vi "OverlayFittedCircle.vi"(10 "Circle time series":dbl[][](array[numeric]), 11 "Image":T1) -> (3 "Image Out":T1)   [LabVIEW 2013]
uses:
  <vilib>/vision/Image Controls.llb/IMAQ Image.ctl
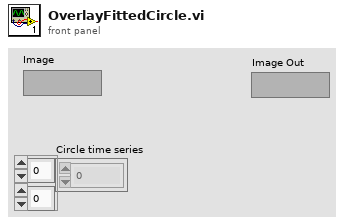
[diagram p1: front panel]
types:
  T1 = typedef "IMAQ Image.ctl" = refnum<image>
  T2 = cluster{"[0]":i32, "[1]":i32, "[2]":i32, "[3]":i32}
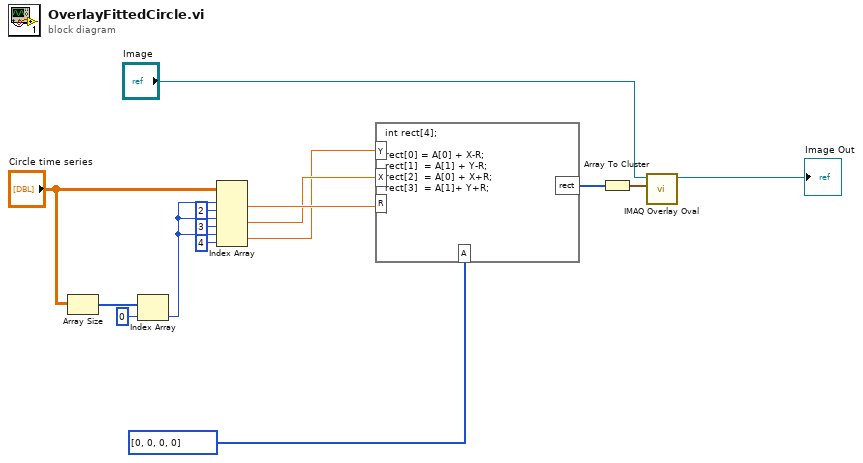
[diagram p0: block diagram]
diagram:
  n1 = Array Size(array="Circle time series") -> (size(s)=w6:i32[])
  n2 = Index Array(array=w6, index=0) -> (element=w4:i32)
  n3 = Index Array(array="Circle time series", index (row) #1=w4, index (col) #1=2 ("disabled index (col)"), index (row) #2=w4, index (col) #2=3 ("disabled index (col)"), index (row) #3=w4, index (col) #3=4 ("disabled index (col)")) -> (element #1=w9:dbl, element #2=w8:dbl, element #3=w7:dbl)
  n4 = formula code="int rect[4];\n\nrect[0] = A[0] + X-R;\nrect[1]  = A[1] + Y-R;\nrect[2]  = A[0] + X+R;\nrect[3]  = A[1]+ Y+R;\n\n;"("X"=w8, "Y"=w7, "R"=w9, "A"=i32[] [0, 0, 0, 0] ("input variable")) -> ("rect"=w14:i32[])
  n5 = Array To Cluster(array=w14) -> (cluster=w15:T2)
  n6 = call "IMAQ Overlay Oval"("Bounding Rectangle"=w15, "Image"="Image") -> ("Image Out"=→"Image Out":T1)  [unwired: 8 in, 1 out]
